vi "Read.vi"(8 "error in (no error)":errorcluster, 10 "TimeOut(s)":dbl, 11 "LT_UpgradeFlash in":refnum<class "LT_UpgradeFlash.lvclass">) -> (0 "error out":errorcluster, 1 "resultStr":string, 2 "ActionResult":bool, 3 "LT_UpgradeFlash out":refnum<class "LT_UpgradeFlash.lvclass">)   [LabVIEW 2017, in "LT_UpgradeFlash.lvclass"]
uses:
  LT_UpgradeFlash.lvclass
  D:/Project/Tymphany/LT_UpgradeFlash/New_Lib/LT_UpgradeFlash_dll/LT_UpgradeFlash_dll/bin/Debug/LT_UpgradeFlash_dll.dll
  New_Lib/LT_UpgradeFlash_dll/LT_UpgradeFlash_dll/bin/Debug/LT_UpgradeFlash_dll.dll
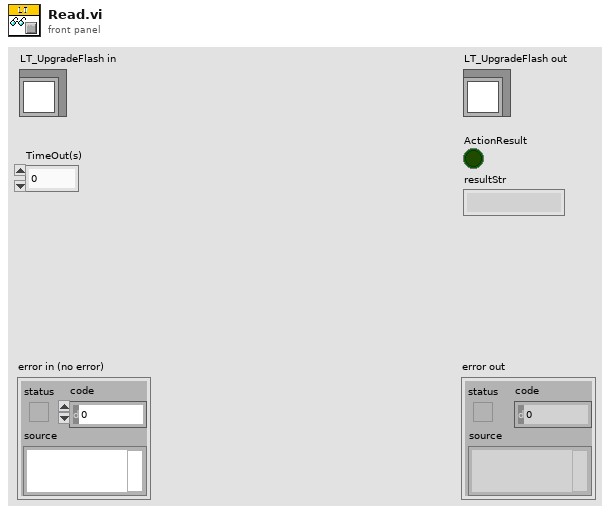
[diagram p1: front panel]
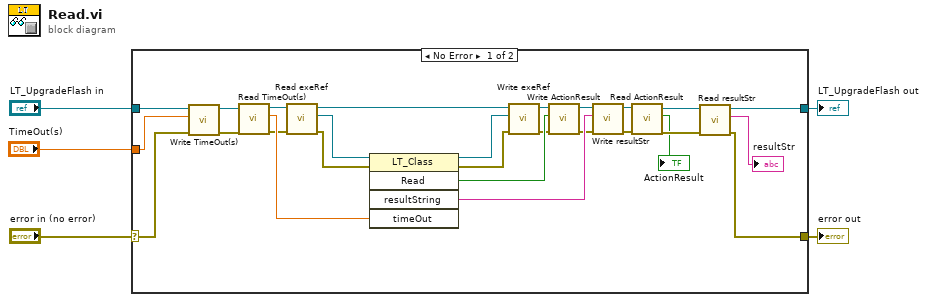
[diagram p0: block diagram]
diagram:
  n1 = case shown="No Error" "error in (no error)" {
    selector: "error in (no error)" -> [w7 w34]
    tunnel: [w11 w34] -> w4
    tunnel: [w12 w33] -> w2
    tunnel: "LT_UpgradeFlash in" -> [w9 w33]
    tunnel: "TimeOut(s)" -> [w6 _]
    frame No Error {
      n2 = call-dynamic "Write TimeOut(s).vi"("error in (no error)"=w7, "TimeOut(s)"=w6, "LT_UpgradeFlash in"=w9) -> ("error out"=w8:errorcluster, "LT_UpgradeFlash out"=w10:refnum<class "LT_UpgradeFlash.lvclass">)  [unwired: 7 in]
      n3 = call-dynamic "Read TimeOut(s).vi"("error in (no error)"=w8, "LT_UpgradeFlash in"=w10) -> ("error out"=w26:errorcluster, "TimeOut(s)"=w31:dbl, "LT_UpgradeFlash out"=w27:refnum<class "LT_UpgradeFlash.lvclass">)  [unwired: 7 in]
      n4 = call-dynamic "Read exeRef.vi"("error in (no error)"=w26, "LT_UpgradeFlash in"=w27) -> ("error out"=w20:errorcluster, "exeRef"=w32:refnum<k24>, "LT_UpgradeFlash out"=w25:refnum<class "LT_UpgradeFlash.lvclass">)  [unwired: 7 in]
      n5 = invoke class="LT_Class" method="Read"(reference=w32, error in=w20, "timeOut"=w31) -> (reference out=w30:refnum<k24>, error out=w19:errorcluster, "Read"=w29:bool, "resultString"=w28:string)  [unwired: 2 in, 1 out]
      n6 = call-dynamic "Write exeRef.vi"("error in (no error)"=w19, "exeRef"=w30, "LT_UpgradeFlash in"=w25) -> ("error out"=w23:errorcluster, "LT_UpgradeFlash out"=w24:refnum<class "LT_UpgradeFlash.lvclass">)  [unwired: 7 in]
      n7 = call-dynamic "Write ActionResult.vi"("error in (no error)"=w23, "ActionResult"=w29, "LT_UpgradeFlash in"=w24) -> ("error out"=w21:errorcluster, "LT_UpgradeFlash out"=w22:refnum<class "LT_UpgradeFlash.lvclass">)  [unwired: 7 in]
      n8 = call-dynamic "Write resultStr.vi"("error in (no error)"=w21, "resultStr"=w28, "LT_UpgradeFlash in"=w22) -> ("error out"=w13:errorcluster, "LT_UpgradeFlash out"=w14:refnum<class "LT_UpgradeFlash.lvclass">)  [unwired: 7 in]
      n9 = call-dynamic "Read ActionResult.vi"("error in (no error)"=w13, "LT_UpgradeFlash in"=w14) -> ("error out"=w17:errorcluster, "ActionResult"=→"ActionResult":bool, "LT_UpgradeFlash out"=w18:refnum<class "LT_UpgradeFlash.lvclass">)  [unwired: 7 in]
      n10 = call-dynamic "Read resultStr.vi"("error in (no error)"=w17, "LT_UpgradeFlash in"=w18) -> ("error out"=w11:errorcluster, "resultStr"=→"resultStr":string, "LT_UpgradeFlash out"=w12:refnum<class "LT_UpgradeFlash.lvclass">)  [unwired: 7 in]
    }
    frame Error {
    }
  }
  "error out" <- w4
  "LT_UpgradeFlash out" <- w2
